vi "Direction Cosines To Euler Angles.vi"(11 "Direction Cosines":dbl[][](array[numeric])) -> (0 "error":i32, 3 "Euler Angles":cluster{"phi":dbl, "theta":dbl, "psi":dbl})   [LabVIEW 2010, in "NI_AALPro.lvlib"]
doc: "Converts a 3-by-3 matrix of direction cosines into Euler angles."
uses:
  NI_AALPro.lvlib
  lvanlys.dll
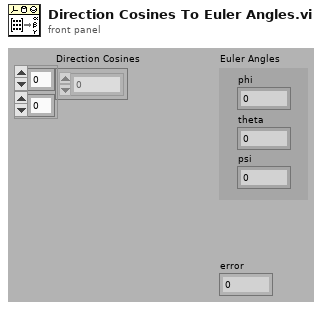
[diagram p1: front panel]
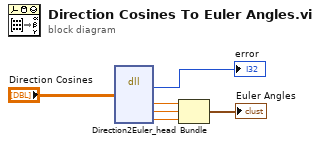
[diagram p0: block diagram]
diagram:
  n1 = dll-call lib="C:/Program Files/National Instruments/LabVIEW 2010/resource/lvanlys.*" fn="Direction2Euler_head"("direction"="Direction Cosines") -> (→"error":i32, "phi"=w4:dbl, "theta"=w3:dbl, "psi"=w2:dbl)  [unwired: 7 in, 2 out]
  n2 = Bundle("phi"=w4, "theta"=w3, "psi"=w2) -> (→"Euler Angles":cluster{"phi":dbl, "theta":dbl, "psi":dbl})  [unwired: 1 in]
